vi "Overlay.vi"(8 "error in (no error)":errorcluster, 10 "Image In":T1, 11 "Overlay Base in":refnum<class "Analyze Results Beam Deviation.lvclass">) -> (0 "error out":errorcluster, 2 "Image out":T1, 3 "Overlay Base out":refnum<class "Analyze Results Beam Deviation.lvclass">)   [LabVIEW 2020, in "Analyze Results Beam Deviation.lvclass"]
uses:
  Analyze Results Beam Deviation.lvclass
  C:/Users/AlexK/work/LabVIEW Programme/POLARIS-AS-3-Cams/Submodules/HIJ Vision/Analyze/Results and Overlays/Results Base/Analyze Results Base.lvclass
  <vilib>/vision/Image Controls.llb/IMAQ Image.ctl
  Analyze Results Beam Deviation.lvclass/Analyze Results Beam Deviation.ctl
  Results Base/Analyze Results Base.lvclass/Analyze Results Base.ctl
  Results Base/Read Overlay_.vi
  Results Base/Read Overlay colors.vi
  Results Base/Read Font, Size & Style.vi
  Results Base/Read Position.vi
  Results Base/Analyze Results Base.lvclass
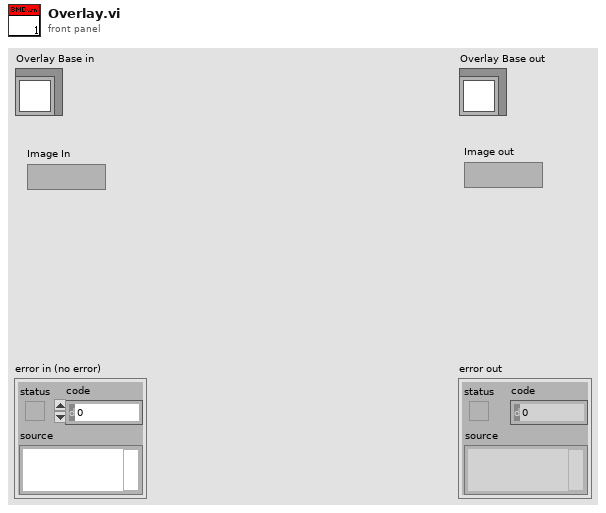
[diagram p1: front panel]
types:
  T1 = typedef "IMAQ Image.ctl" = refnum<image>
  T2 = cluster{"Desired Font (Application)":enum16{"User-specified Font", "Application Font", "System Font", "Dialog Font"}, "[User-specified Font]":cluster{"Font Name":string, "Size":i16, "Strikeout?":bool, "Italic?":bool, "Underline?":bool, "Outline?":bool, "Shadow?":bool, "Bold?":bool, "Rotation Angle":dbl}, "Horizontal Alignment":i16, "Vertical Alignment":i16}
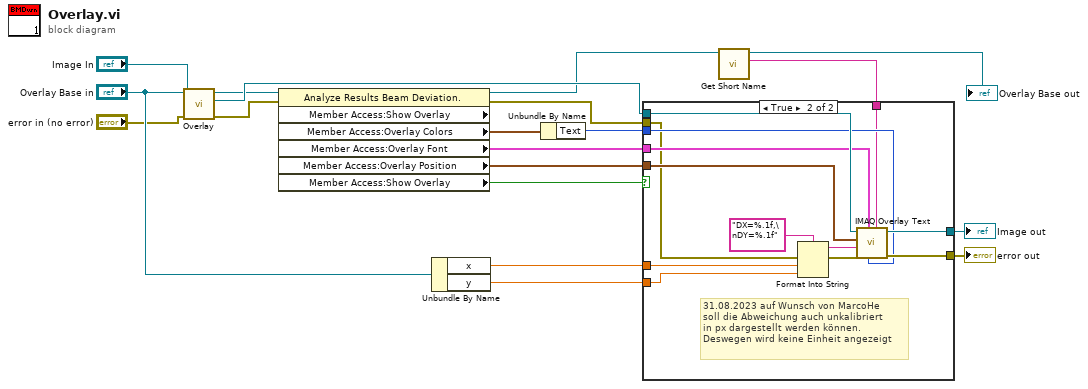
[diagram p0: block diagram]
diagram:
  n1 = call-parent "Overlay.vi"("error in (no error)"="error in (no error)", "Image In"="Image In", "Overlay Base in"="Overlay Base in") -> ("error out"=w5:errorcluster, "Image out"=w16:T1, "Overlay Base out"=w7:refnum<class "Analyze Results Beam Deviation.lvclass">)  [unwired: 6 in]
  n2 = property class="Analyze Results Beam Deviation." props=["Member Access:Show Overlay", "Member Access:Overlay Colors", "Member Access:Overlay Font", "Member Access:Overlay Position", "Member Access:Show Overlay"](reference=w7, error in=w5) -> (reference out=w3:refnum<class "Analyze Results Beam Deviation.lvclass">, error out=w4:errorcluster, "Member Access:Overlay Colors"=w13:cluster{"Border":u32, "Text":u32}, "Member Access:Overlay Font"=w11:T2, "Member Access:Overlay Position"=w10:cluster{"x":i16, "y":i16}, "Member Access:Show Overlay"=w9:bool)  [unwired: 1 out]
  n3 = Unbundle By Name("Overlay Base in") -> ("x"=w15:sgl, "y"=w14:sgl)
  n4 = Unbundle By Name(w13) -> ("Text"=w12:u32)
  n5 = call-dynamic "Get Short Name.vi"("Analyze Results Base in"=w3) -> ("Short Name"=w1:string, "Analyze Results Base out"=→"Overlay Base out":refnum<class "Analyze Results Beam Deviation.lvclass">)  [unwired: 8 in, 1 out]
  n6 = case shown="True" w9 {
    tunnel: w16 -> [w21 w34]
    tunnel: [w21 w33] -> w17
    tunnel: [w20 w32] -> w18
    tunnel: w4 -> [w20 w26]
    tunnel: w15 -> [_ w28]
    tunnel: w14 -> [_ w27]
    tunnel: w12 -> [_ w31]
    tunnel: w11 -> [_ w30]
    tunnel: w10 -> [_ w29]
    tunnel: w1 -> [_ w22]
    frame False {
    }
    frame True {
      # "31.08.2023 auf Wunsch von MarcoHe\nsoll die Abweichung auch unkalibriert\nin px dargestellt werden können.\nDeswegen wird keine Einheit angezeigt"
      n7 = Format Into String(format string="DX=%.1f,\nDY=%.1f", error in=w26, w28, w27) -> (resulting string=w25:string, error out=w24:errorcluster)  [unwired: 1 in]
      n8 = call "IMAQ Overlay Text"("Group"=w22, "Text Color (black)"=w31, "Font, Size & Style"=w30, "error in (no error)"=w24, "String"=w25, "Origin"=w29, "Image"=w34) -> ("error out"=w32:errorcluster, "Image Out"=w33:T1)  [unwired: 3 in]
    }
  }
  "error out" <- w18
  "Image out" <- w17
